vi "NF WF1973_74 SQU Ext.vi"(6 "Read(F)":bool, 8 "error in (no error)":errorcluster caption="Error IN", 9 "Extend(OFF)":bool, 10 "Ch(Ch1)":bool, 11 "VISAsession":refnum<visa-resource-name>) -> (0 "error out":errorcluster caption="Error OUT", 2 "Query State":i32, 3 "CopyVISAsession":refnum<visa-resource-name>)   [LabVIEW 2010]
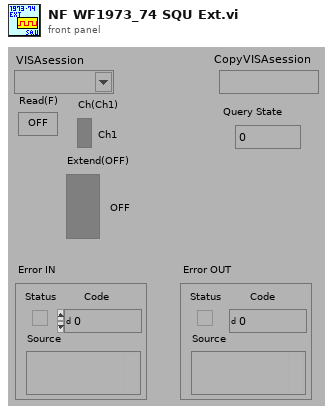
[diagram p1: front panel]
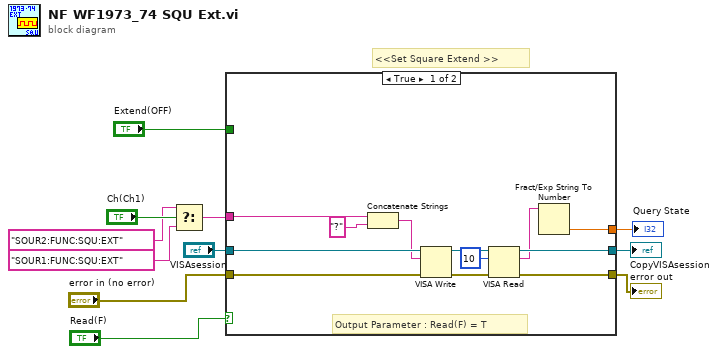
[diagram p0: block diagram]
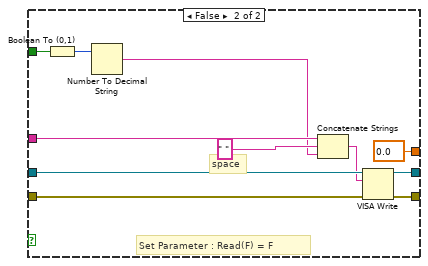
[diagram p2: hidden frame]
diagram:
  # "<<Set Square Extend >>"
  n1 = Select(t="SOUR2:FUNC:SQU:EXT" ("文字列"), s="Ch(Ch1)", f="SOUR1:FUNC:SQU:EXT" ("文字列")) -> (s? t:f=w4:string)
  n2 = case shown="TRUE" "Read(F)" {
    tunnel: "VISAsession" -> [w23 w34]
    tunnel: [w20 w32] -> w10
    tunnel: [w19 w33] -> w9
    tunnel: "error in (no error)" -> [w18 w28]
    tunnel: w4 -> [w16 w29]
    tunnel: [w12 0.0] -> w6
    tunnel: "Extend(OFF)" -> [_ w26]
    frame True {
      # "Output Parameter : Read(F) = T"
      n3 = Concatenate Strings(w16, "?" ("形式文字列")) -> (w14:string)
      n4 = VISA Write(VISA resource name=w23, write buffer=w14, error in (no error)=w18) -> (VISA resource name out=w21:refnum<visa-resource-name>, error out=w22:errorcluster)  [unwired: 1 out]
      n5 = VISA Read(VISA resource name=w21, byte count=u32 10 ("バイトカウント（0）"), error in (no error)=w22) -> (VISA resource name out=w20:refnum<visa-resource-name>, read buffer=w13:string, error out=w19:errorcluster)  [unwired: 1 out]
      n6 = Fract/Exp String To Number(string=w13) -> (number=w12:dbl)  [unwired: 3 in, 1 out]
    }
    frame False {
      # "space"
      # "Set Parameter : Read(F) = F"
      n7 = Boolean To (0,1)(Boolean=w26) -> (0, 1=w25:i16)
      n8 = Number To Decimal String(number=w25) -> (decimal integer string=w24:string)  [unwired: 1 in]
      n9 = Concatenate Strings(w29, " ", w24) -> (w31:string)
      n10 = VISA Write(VISA resource name=w34, write buffer=w31, error in (no error)=w28) -> (VISA resource name out=w32:refnum<visa-resource-name>, error out=w33:errorcluster)  [unwired: 1 out]
    }
  }
  "error out" <- w9
  "CopyVISAsession" <- w10
  "Query State" <- w6
